vi "GSP_Manager_TCSLINK_handler.vi"(4 "error in (no error)":errorcluster, 6 "Actions":T1) -> (0 "error out":errorcluster, 2 "reference out (launch only)":refnum<vi>)   [LabVIEW 2015]
uses:
  TCSLINK_handler_actions.ctl
  SystemUtil/Command.ctl
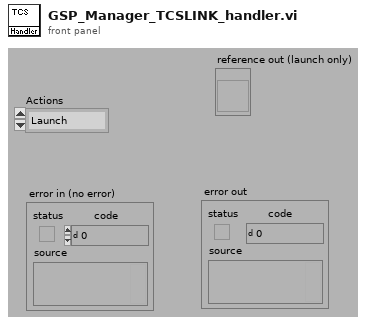
[diagram p1: front panel]
types:
  T1 = typedef "TCSLINK_handler_actions.ctl" = enum16{"Launch", "Shutdown"}
  T2 = typedef "Command.ctl" = cluster{"Command":string, "Parameter":string}
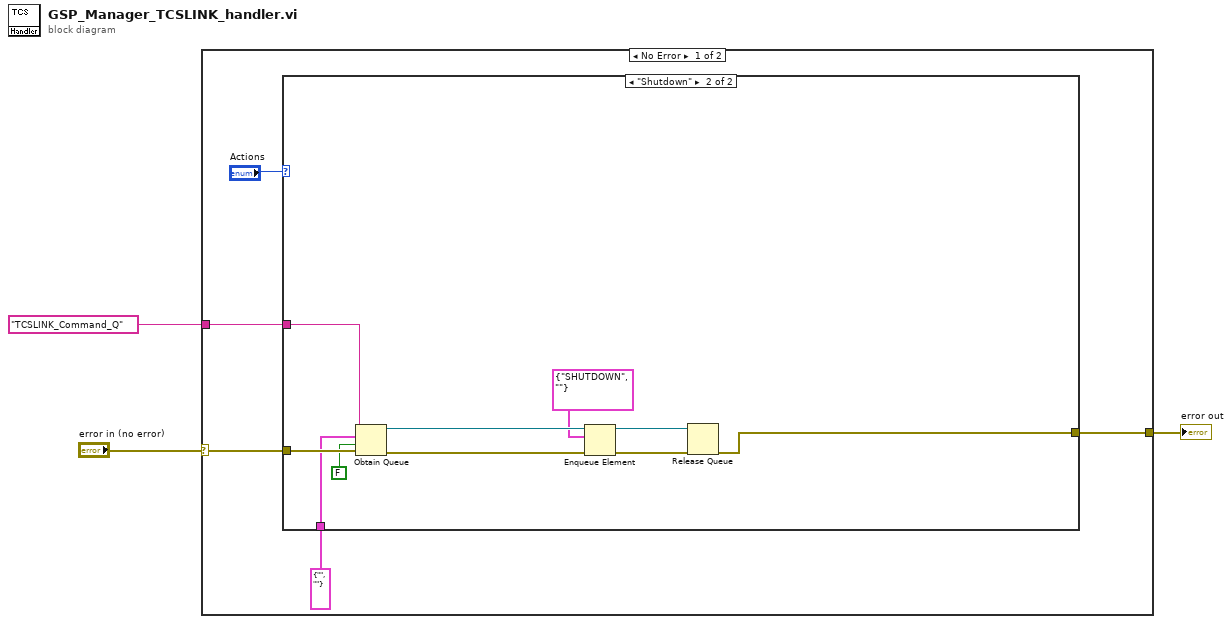
[diagram p0: block diagram]
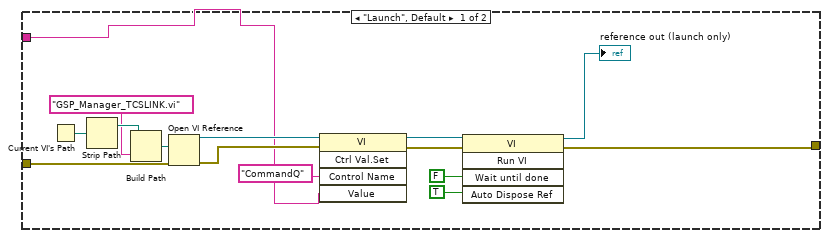
[diagram p2: hidden frame]
diagram:
  n1 = case shown="No Error" "error in (no error)" {
    selector: "error in (no error)" -> [w5 w34]
    tunnel: [w8 w34] -> w3
    tunnel: "TCSLINK_Command_Q" -> [w7 _]
    frame No Error {
      n2 = case shown="\"Shutdown\"" "Actions" {
        tunnel: w5 -> [w23 w33]
        tunnel: [w16 w24] -> w8
        tunnel: w7 -> [w9 w31]
        tunnel: T2 {"Command"="", "Parameter"=""} ("Command") -> [_ w28]
        frame "Launch", Default {
          n3 = Current VI's Path() -> (path=w20:path)
          n4 = Strip Path(path=w20) -> (stripped path=w18:path)  [unwired: 1 out]
          n5 = Build Path(base path=w18, name or relative path="GSP_Manager_TCSLINK.vi" ("vi path")) -> (appended path=w19:path)
          n6 = Open VI Reference(vi path=w19, error in (no error)=w23) -> (vi reference=w12:refnum<vi>, error out=w11:errorcluster)  [unwired: 4 in]
          n7 = invoke class="VI" method="Ctrl Val.Set"(reference=w12, error in=w11, "Control Name"="CommandQ", "Value"=w9) -> (reference out=w14:refnum<vi>, error out=w13:errorcluster)  [unwired: 1 in, 3 out]
          n8 = invoke class="VI" method="Run VI"(reference=w14, error in=w13, "Wait until done"=FALSE, "Auto Dispose Ref"=TRUE) -> (reference out=→"reference out (launch only)":refnum<vi>, error out=w16:errorcluster)  [unwired: 1 in, 3 out]
        }
        frame "Shutdown" {
          n9 = Obtain Queue(name (unnamed)=w31, element data type=w28, create if not found? (T)=FALSE, error in (no error)=w33) -> (queue out=w30:refnum<queue>, error out=w32:errorcluster)  [unwired: 1 in, 1 out]
          n10 = Enqueue Element(queue=w30, element=T2 {"Command"="SHUTDOWN", "Parameter"=""}, error in (no error)=w32) -> (queue out=w26:refnum<queue>, error out=w25:errorcluster)  [unwired: 1 in, 1 out]
          n11 = Release Queue(queue=w26, error in (no error)=w25) -> (error out=w24:errorcluster)  [unwired: 1 in, 2 out]
        }
      }
    }
    frame Error {
    }
  }
  "error out" <- w3
